vi "KM_ControlHFLI -- V4.vi.vi"(4 "Control HFLI command":T2=enum."Scan frequency", 8 "ZI HFLI System Parameters IN":T1={"IP Address"="DEV3523", "Start (Hz)"=44300.0, "Stop (Hz)"=44600.0, "Filter Order"=4, "Number of Points"=100, "Precision"=0, "Bandwidth (Hz)"=50.0, "Averaging"=1, "Log Sweep"=FALSE, "Demod"=0} {"Averaging" items=["1"=1, "2"=2, "4"=4, "16"=16, "32"=32, "64"=64]; "Bandwidth (Hz)" format="%#_p"; "Precision" items=["Low", "Med", "High"]; "Number of Points" min=2 max=66000; "Filter Order" items=["6, 1st"=1, "12, 2nd"=2, "18, 3rd"=3, "24, 4th"=4, "30, 5th"=5, "36, 6th"=6, "42, 7th"=7, "48, 8th"=8]; "Stop (Hz)" format="%_5p"; "Start (Hz)" format="%_5p"}) -> (0 "Voltage out":cdb[](array[numeric]), 1 "Freq out":dbl[](array[numeric]), 3 "ZI HFLI System Parameters OUT":T1={"IP Address"="DEV3523", "Start (Hz)"=44300.0, "Stop (Hz)"=44.7, "Filter Order"=4, "Number of Points"=100, "Precision"=0, "Bandwidth (Hz)"=50.0, "Averaging"=1, "Log Sweep"=FALSE, "Demod"=0} {"Averaging" items=["1"=1, "2"=2, "4"=4, "16"=16, "32"=32, "64"=64]; "Bandwidth (Hz)" format="%#_p"; "Precision" items=["Low", "Med", "High"]; "Number of Points" min=2 max=66000; "Filter Order" items=["6, 1st"=1, "12, 2nd"=2, "18, 3rd"=3, "24, 4th"=4, "30, 5th"=5, "36, 6th"=6, "42, 7th"=7, "48, 8th"=8]; "Stop (Hz)" format="%_5p"; "Start (Hz)" format="%_5p"})   [LabVIEW 2016]
doc: "Control a Zurich instrument device via the LabOne Labview API. \nRequirements: Zurich Instruments HF2 (HF2IS or HF2LI-MF ).\nThis example uses the API functions to perform a frequency sweep and measure the impedance. \n\n© Zurich Instruments AG, www.zhinst.com"
uses:
  KM_ControlHFLIcommand.ctl
  KM_SystemParameters.ctl
panel:
  out "cal_types":cluster{string[], bool[]}[](array[cluster])=[{["R (Ohms)", " ", " "], [TRUE, FALSE, FALSE]}, {["C (F)", " ", " "], [TRUE, FALSE, FALSE]}, {["L (H)", " ", " "], [TRUE, FALSE, FALSE]}, {["R (Ohms)", "C (F)\n ", " "], [TRUE, TRUE, FALSE]}]
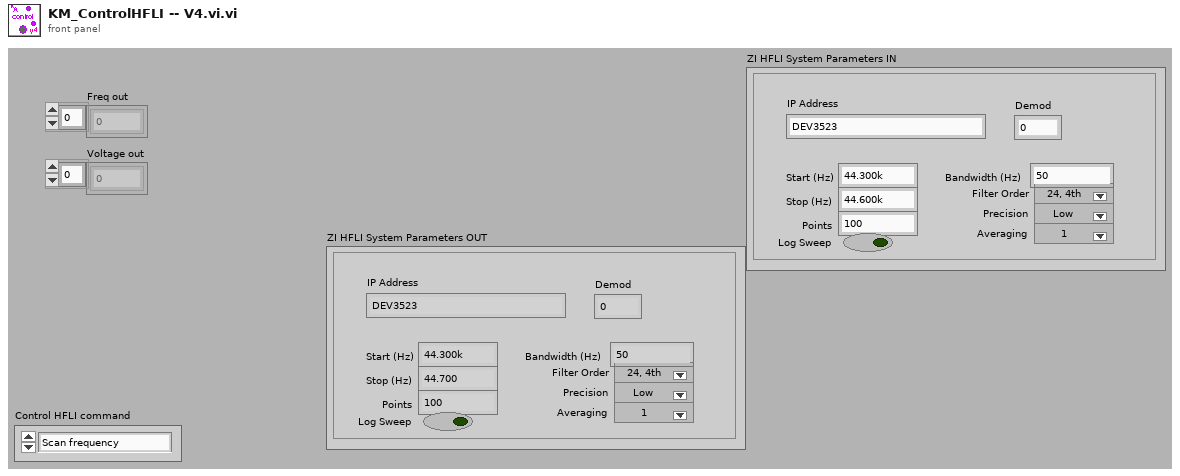
[diagram p1: front panel]
types:
  T1 = typedef "KM_SystemParameters.ctl" = cluster{"IP Address":string, "Start (Hz)":dbl, "Stop (Hz)":dbl, "Filter Order":i32, "Number of Points":i32, "Precision":u16, "Bandwidth (Hz)":dbl, "Averaging":u16, "Log Sweep":bool, "Demod":i32}
  T2 = typedef "KM_ControlHFLIcommand.ctl" = enum16{"Initialize", "Scan frequency"}
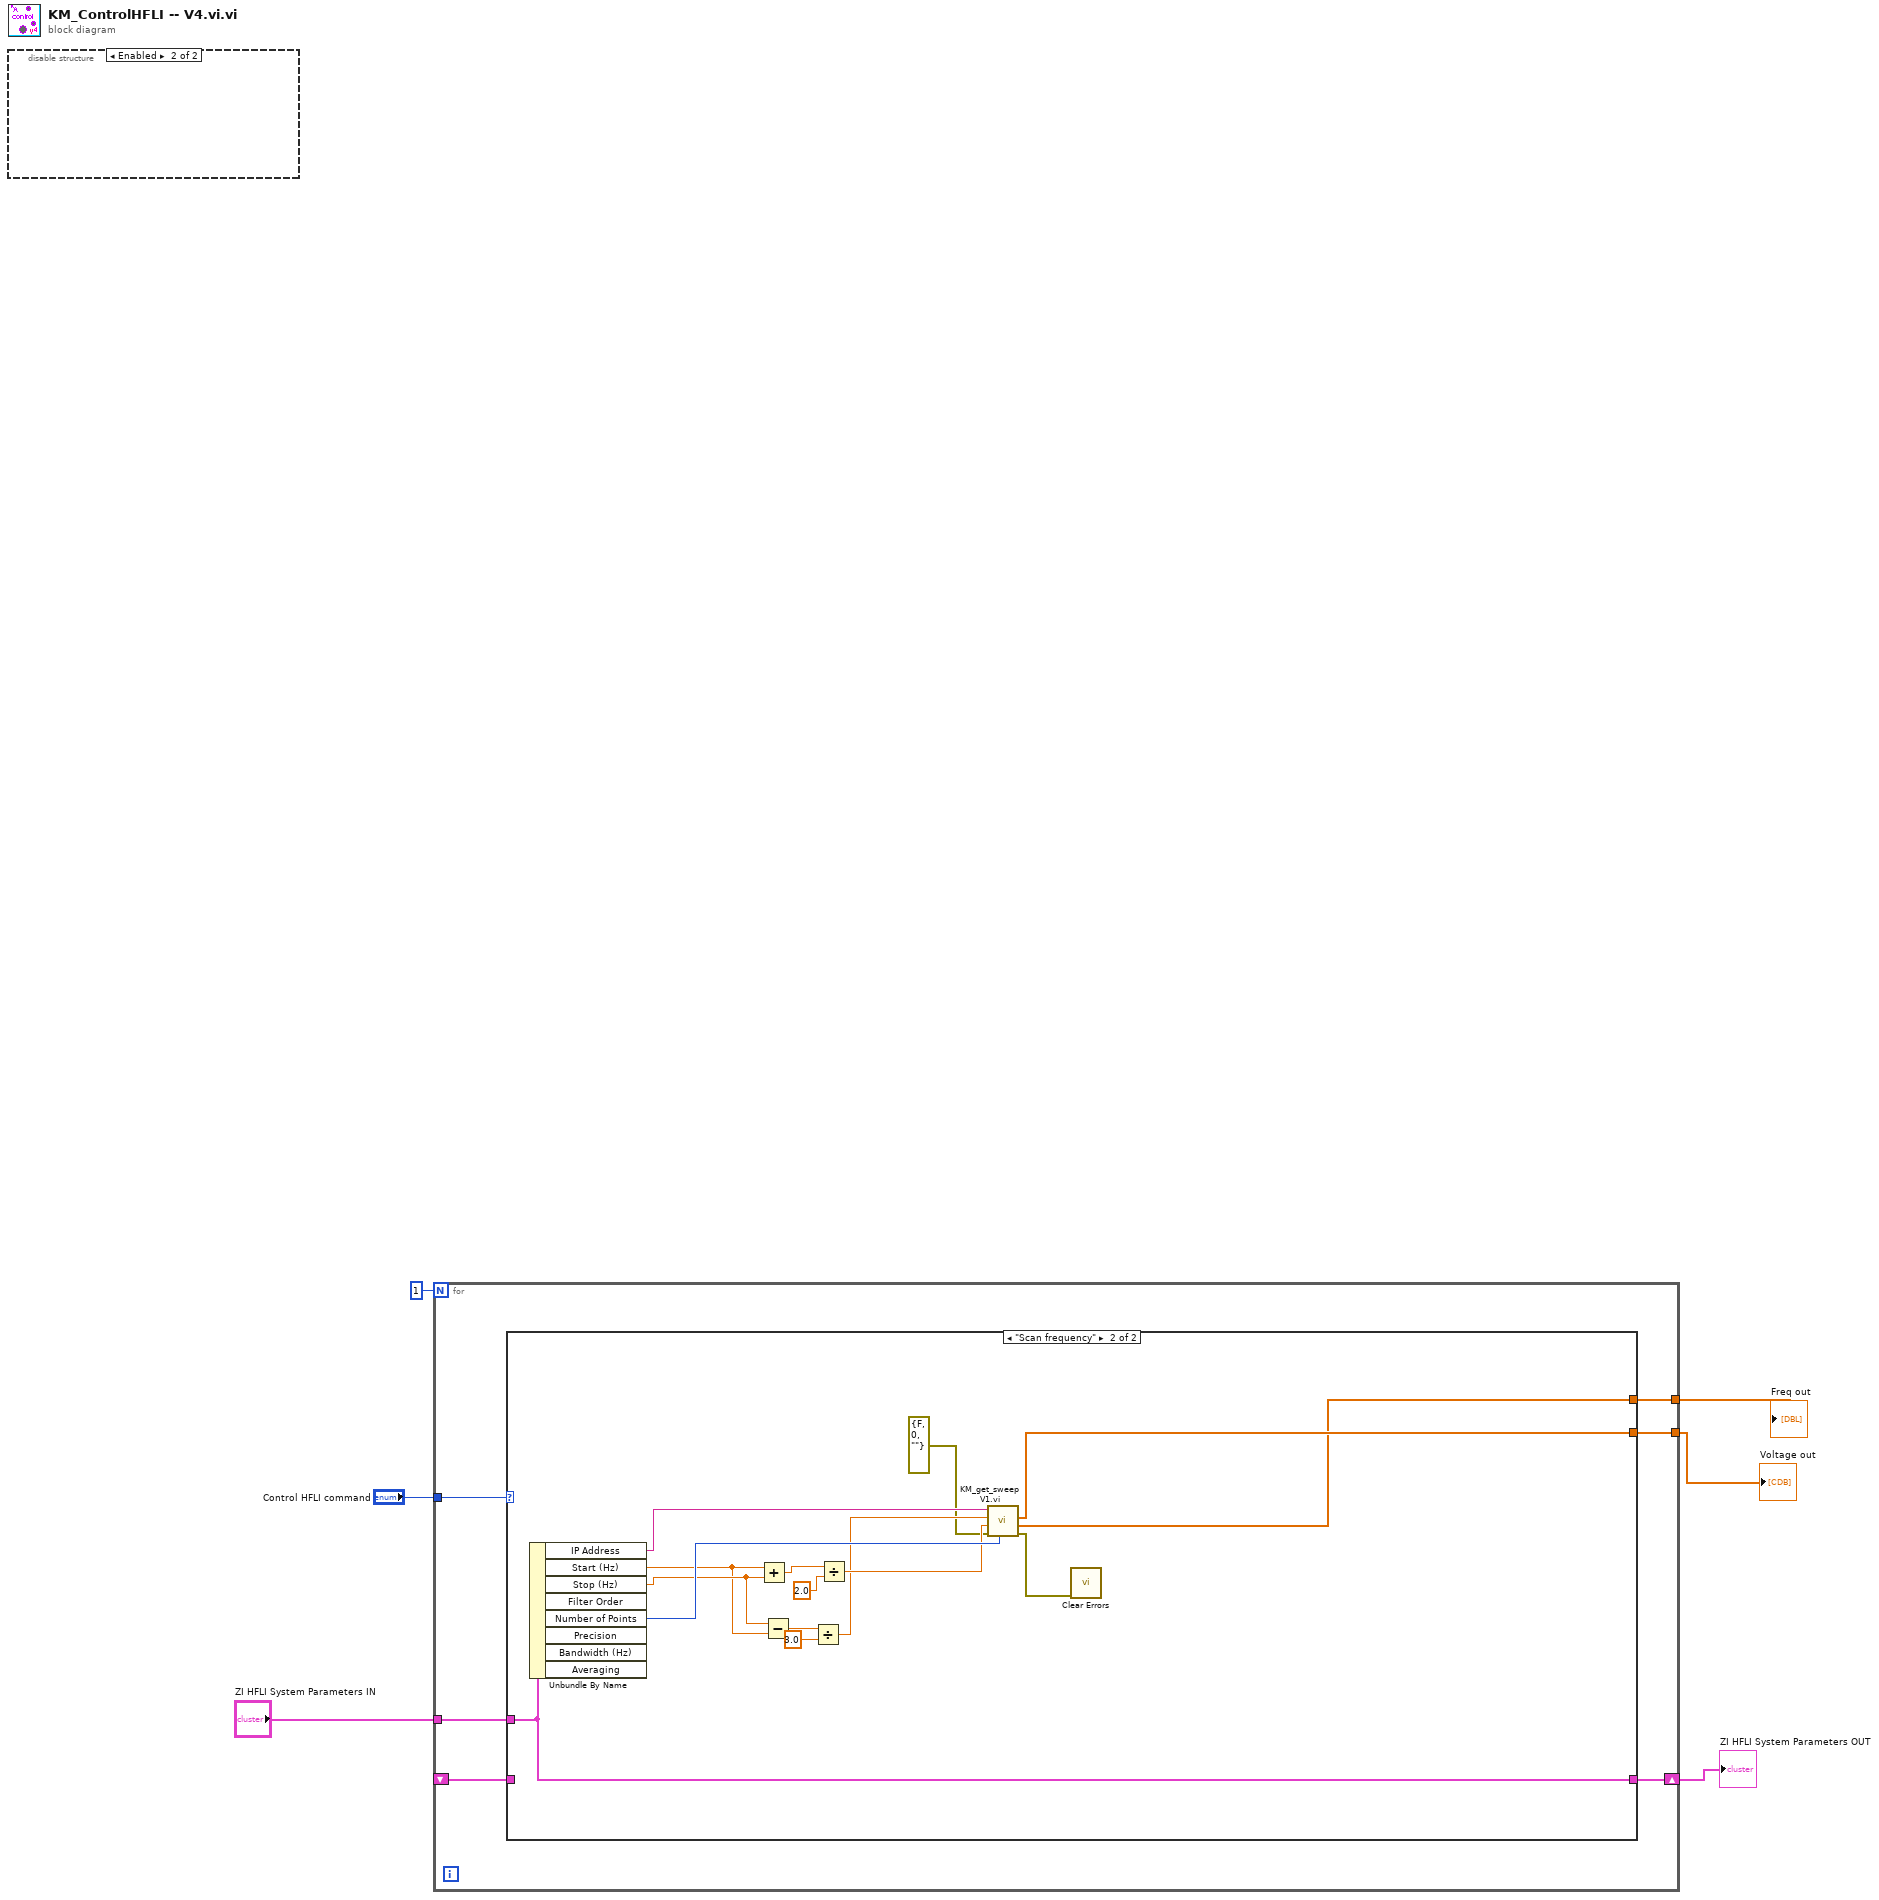
[diagram p0: block diagram]
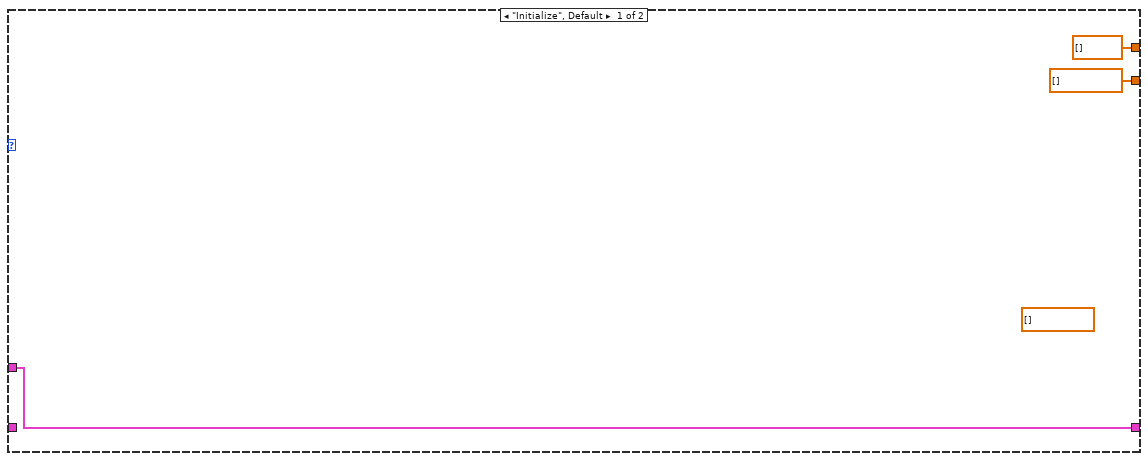
[diagram p2: hidden frame]
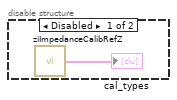
[diagram p3: hidden frame]
diagram:
  n1 = disable-structure shown="Enabled" {
    frame Disabled {
      n2 = call "ziImpedanceCalibRefZ.vi"() -> ("cal_types"=→"cal_types":cluster{string[], bool[]}[], 2:w7)  [unwired: 3 in, 1 out]
    }
    frame Enabled {
    }
  }
  n3 = for {
    N: 1 -> [_]
    tunnel: "Control HFLI command" -> [w14]
    tunnel: "ZI HFLI System Parameters IN" -> [w13]
    shift-right: [w12] -> w2
    shift-left: _ -> [w11]
    tunnel: [w10] -> w4
    tunnel: [w9] -> w3
    n4 = case shown="\"Scan frequency\"" w14 {
      tunnel: w13 -> [w17 w18]
      tunnel: [w17 w18] -> w12
      tunnel: w11 -> [_ _]
      tunnel: [dbl[] [] w21] -> w10
      tunnel: [cdb[] [] w22] -> w9
      frame "Initialize", Default {
        (unwired) cdb[] []
      }
      frame "Scan frequency" {
        n5 = Unbundle By Name(w18) -> ("IP Address"=w31:string, "Start (Hz)"=w26:dbl, "Stop (Hz)"=w27:dbl, "Number of Points"=w32:i32)  [unwired: 4 out]
        n6 = Add(x=w26, y=w27) -> (x+y=w30:dbl)
        n7 = Subtract(x=w27, y=w26) -> (x-y=w25:dbl)
        n8 = Divide(x=w25, y=3.0) -> (x/y=w23:dbl)
        n9 = Divide(x=w30, y=2.0) -> (x/y=w28:dbl)
        n10 = call "KM_get_sweep V1.vi.vi"("N"=w32, "Error In"=errorcluster {"status"=FALSE, "code"=0, "source"=""}, "omega0 (Hz)"=w28, "gamma (Hz)"=w23, "Address"=w31) -> ("Error Out"=w19:errorcluster, "freq out (Hz)"=w21:dbl[], "voltage out (V)"=w22:cdb[])  [unwired: 4 in]
        n11 = call <vilib>:"Clear Errors.vi"("error in (no error)"=w19) -> ()  [unwired: 5 in, 2 out]
      }
    }
  }
  "Freq out" <- w4
  "Voltage out" <- w3
  "ZI HFLI System Parameters OUT" <- w2
